vi "WILT Build Array of Start Buttons and Water Valves.vi"(8 "Error In":errorcluster, 10 "Agilent Valve and Switch Locations":T1[](array[typedef]), 11 "Label Search":string) -> (0 "Error Out":errorcluster, 3 "Array of Values":string[][](array[string]))   [LabVIEW 2016]
uses:
  Type Definitions/WILT Agilent Channel Definition.ctl
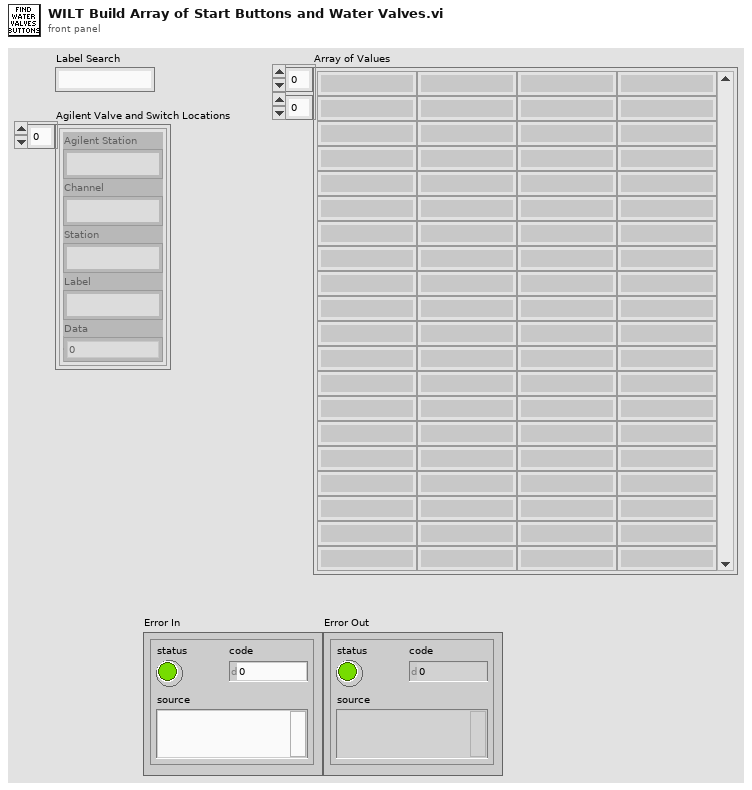
[diagram p1: front panel]
types:
  T1 = typedef "WILT Agilent Channel Definition.ctl" = cluster{"Channel":string, "Station":string, "Label":string, "Agilent Station":string, "Data":dbl}
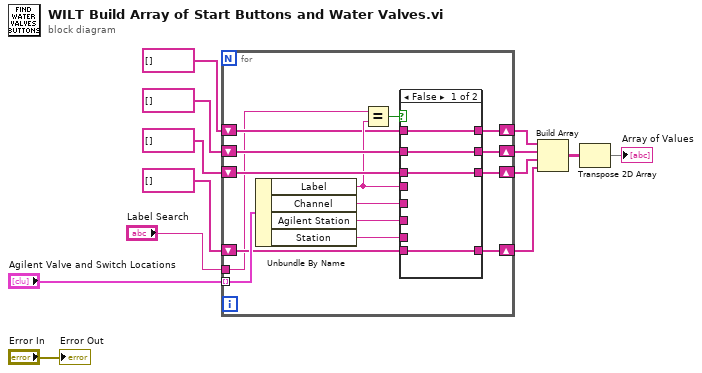
[diagram p0: block diagram]
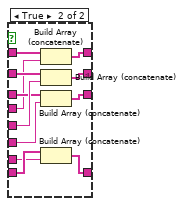
[diagram p2: hidden frame]
diagram:
  n1 = for {
    tunnel: "Agilent Valve and Switch Locations" -> [w28] mode=indexing
    shift-right: [w24] -> w6
    shift-left: string[] [] -> [w26]
    shift-right: [w21] -> w7
    shift-left: string[] [] -> [w22]
    shift-right: [w19] -> w8
    shift-left: string[] [] -> [w20]
    shift-right: [w15] -> w12
    shift-left: string[] [] -> [w16]
    tunnel: "Label Search" -> [w14]
    n2 = Unbundle By Name(w28) -> ("Label"=w17:string, "Channel"=w25:string, "Agilent Station"=w23:string, "Station"=w18:string)
    n3 = Equal?(x=w14, y=w17) -> (x = y?=w27:bool)
    n4 = case shown="False" w27 {
      tunnel: w26 -> [w32 w44]
      tunnel: w25 -> [_ w43]
      tunnel: [w32 w42] -> w24
      tunnel: w23 -> [_ w39]
      tunnel: w22 -> [w31 w41]
      tunnel: [w31 w40] -> w21
      tunnel: w20 -> [w30 w38]
      tunnel: [w30 w37] -> w19
      tunnel: w18 -> [_ w36]
      tunnel: w17 -> [_ w35]
      tunnel: w16 -> [w29 w34]
      tunnel: [w29 w33] -> w15
      frame False {
      }
      frame True {
        n5 = Build Array (concatenate)(w34, w35) -> (w33:string[])
        n6 = Build Array (concatenate)(w44, w43) -> (w42:string[])
        n7 = Build Array (concatenate)(w41, w39) -> (w40:string[])
        n8 = Build Array (concatenate)(w38, w36) -> (w37:string[])
      }
    }
  }
  n9 = Build Array(w12, w6, w7, w8) -> (w9:string[][])
  n10 = Transpose 2D Array(2D array=w9) -> (transposed array=→"Array of Values":string[][])
  "Error Out" <- "Error In"
